vi "GetNumberArgument.vi"(1 "Argument":string, 2 "Argument List In":string[](array[string])) -> (0 "value":dbl)   [LabVIEW 2011]
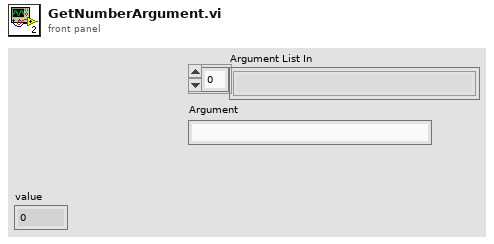
[diagram p1: front panel]
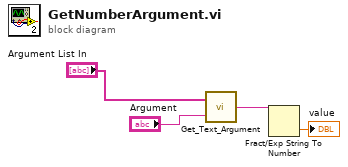
[diagram p0: block diagram]
diagram:
  n1 = call "Get_Text_Argument.vi"("Argument"="Argument", "Argument List"="Argument List In") -> ("Text"=w4:string)
  n2 = Fract/Exp String To Number(string=w4) -> (number=→"value":dbl)  [unwired: 3 in, 1 out]
